vi "Create Log Path.vi"() -> (3 "log path":path)   [LabVIEW 2021, in "Log.lvlib"]
uses:
  Log.lvlib
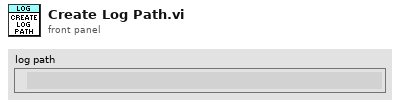
[diagram p1: front panel]
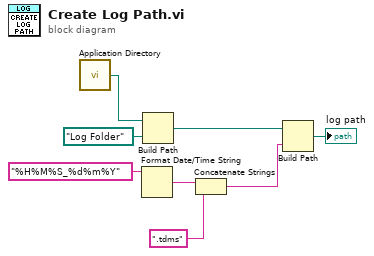
[diagram p0: block diagram]
diagram:
  n1 = call <vilib>:"Application Directory.vi"() -> ("Application Directory"=w7:path)
  n2 = Format Date/Time String(time format string (%c)="%H%M%S_%d%m%Y") -> (date/time string=w4:string)  [unwired: 2 in]
  n3 = Build Path(base path=w7, name or relative path=path "Log Folder") -> (appended path=w5:path)
  n4 = Concatenate Strings(w4, ".tdms" ("string")) -> (w2:string)
  n5 = Build Path(base path=w5, name or relative path=w2) -> (appended path=→"log path":path)
